vi "GetVIParam.vi"(2 "Tipo":T1) -> (16 "vi reference":refnum<vi>)   [LabVIEW 2017]
uses:
  Typedefs/Tipo_TipoSinalSimulado.ctl
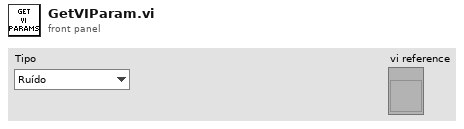
[diagram p1: front panel]
types:
  T1 = typedef "Tipo_TipoSinalSimulado.ctl" = enum16{"Ruído", "Fasor", "Senóide", "Composto", "AM", "Proximidade", "Entreferro"}
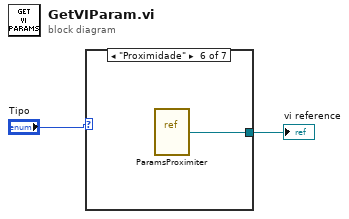
[diagram p0: block diagram]
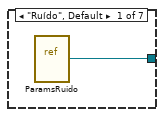
[diagram p2: hidden frame]
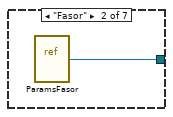
[diagram p3: hidden frame]
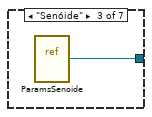
[diagram p4: hidden frame]
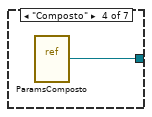
[diagram p5: hidden frame]
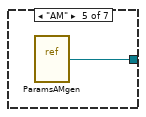
[diagram p6: hidden frame]
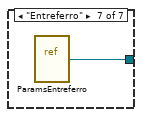
[diagram p7: hidden frame]
diagram:
  n1 = case shown="\"Proximidade\"" "Tipo" {
    tunnel: [w3 w4 w5 w6 w7 w8 w9] -> w1
    frame "Ruído", Default {
      n2 = vi-ref "ParamsRuido.vi"() -> (w3:refnum<vi>)
    }
    frame "Fasor" {
      n3 = vi-ref "ParamsFasor.vi"() -> (w4:refnum<vi>)
    }
    frame "Senóide" {
      n4 = vi-ref "ParamsSenoide.vi"() -> (w5:refnum<vi>)
    }
    frame "Composto" {
      n5 = vi-ref "ParamsComposto.vi"() -> (w6:refnum<vi>)
    }
    frame "AM" {
      n6 = vi-ref "ParamsAMgen.vi"() -> (w7:refnum<vi>)
    }
    frame "Proximidade" {
      n7 = vi-ref "ParamsProximiter.vi"() -> (w8:refnum<vi>)
    }
    frame "Entreferro" {
      n8 = vi-ref "ParamsEntreferro.vi"() -> (w9:refnum<vi>)
    }
  }
  "vi reference" <- w1
